vi "CollimationLightScanOffset.vi"(0 "X Pos Num":i32, 1 "状态":enum16{"计算总分辨率", "计算偏移量"}(ring), 5 "Y Pos Num":i32, 9 "当前X位置":i32, 11 "当前Y位置":i32, 12 "正序？":bool) -> (6 "X Resolution":i32, 10 "Y Resolution":i32, 15 "offset":i32[](array[numeric]))   [LabVIEW 2018]
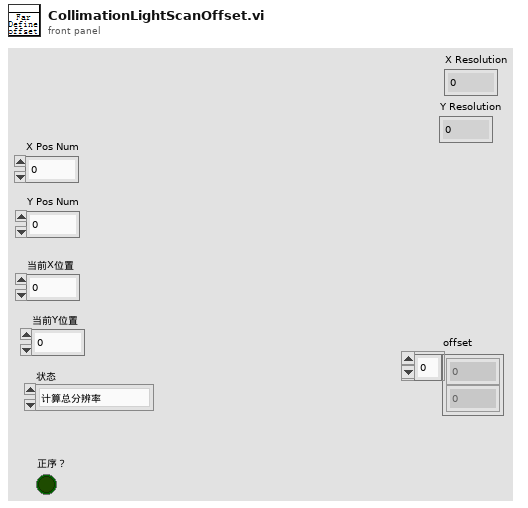
[diagram p1: front panel]
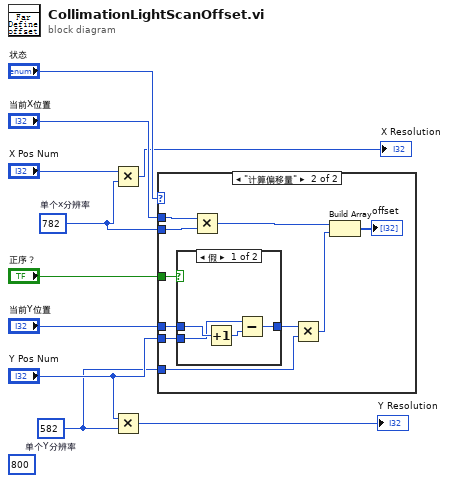
[diagram p0: block diagram]
diagram:
  w2 = 582  # 单个Y分辨率
  w1 = 782  # 单个x分辨率
  (unwired) 800
  n1 = Multiply(x="X Pos Num", y=w1) -> (x*y=→"X Resolution":i32)
  n2 = Multiply(x="Y Pos Num", y=w2) -> (x*y=→"Y Resolution":i32)
  n3 = case shown="\"计算偏移量\"" "状态" {
    tunnel: "Y Pos Num" -> [_ w19]
    tunnel: "当前X位置" -> [_ w15]
    tunnel: "当前Y位置" -> [_ w14]
    tunnel: "正序？" -> [_ w13]
    tunnel: w2 -> [_ w12]
    tunnel: w1 -> [_ w11]
    frame "计算总分辨率", Default {
    }
    frame "计算偏移量" {
      n4 = case shown="假" w13 {
        tunnel: w14 -> [w24 w25]
        tunnel: [w21 w25] -> w20
        tunnel: w19 -> [w23 _]
        frame False {
          n5 = Increment(x=w24) -> (x+1=w22:i32)
          n6 = Subtract(x=w23, y=w22) -> (x-y=w21:i32)
        }
        frame True {
        }
      }
      n7 = Multiply(x=w15, y=w11) -> (x*y=w17:i32)
      n8 = Multiply(x=w20, y=w12) -> (x*y=w16:i32)
      n9 = Build Array(w17, w16) -> (→"offset":i32[])
    }
  }
